vi "Volumes calculation.vi"(1 "Ring":u16(ring) items=["Random", "Regular", "Piecewise regular", "DiRect"], 2 "Params":sgl[][](array[numeric])) -> (0 "Volumes":sgl[](array[numeric]))   [LabVIEW 2018]
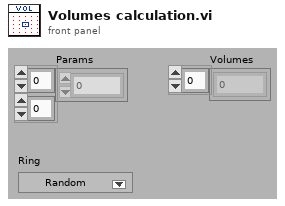
[diagram p1: front panel]
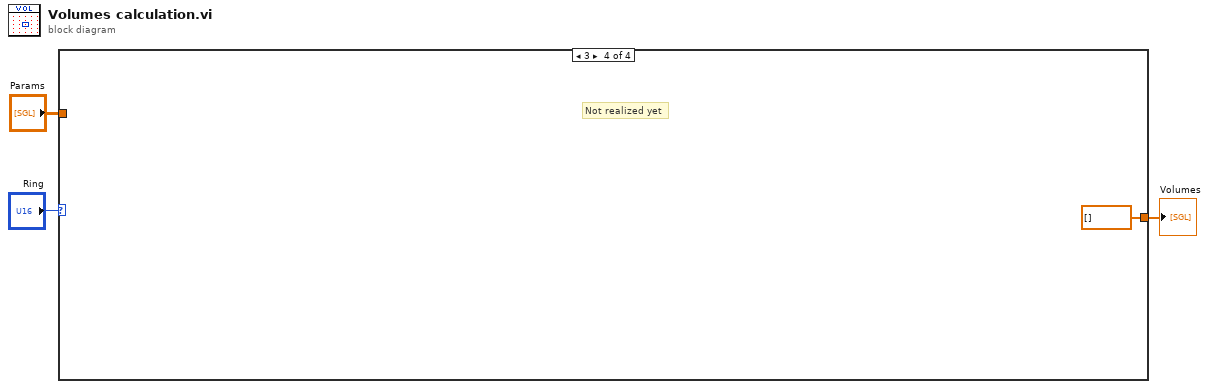
[diagram p0: block diagram]
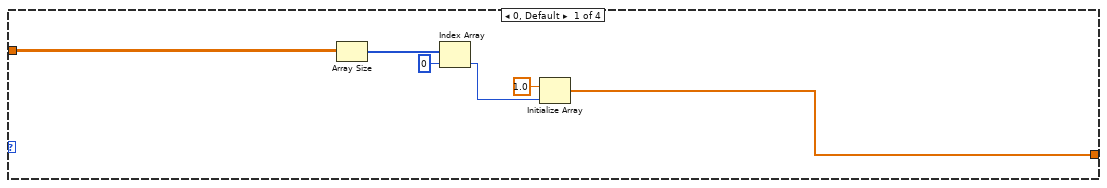
[diagram p2: hidden frame]
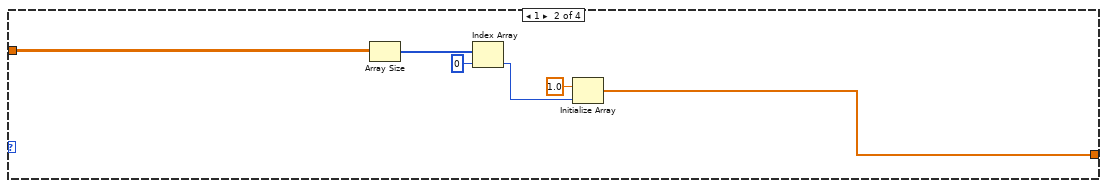
[diagram p3: hidden frame]
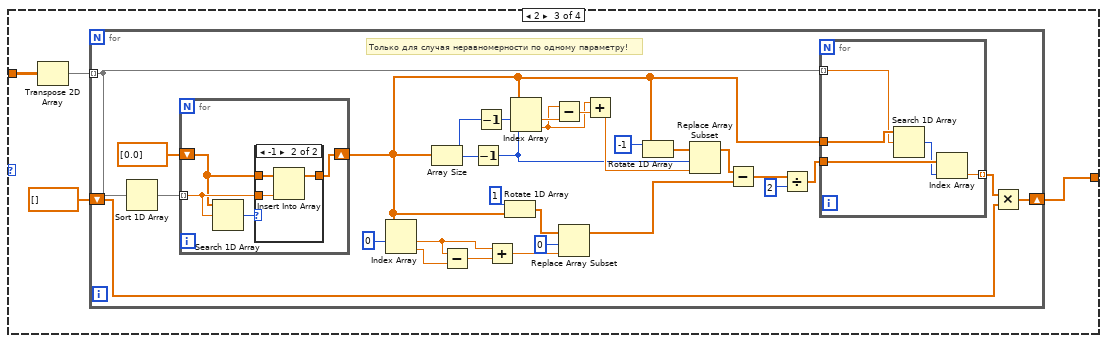
[diagram p4: hidden frame]
diagram:
  n1 = case shown="3" "Ring" {
    tunnel: "Params" -> [w9 w11 w19 _]
    tunnel: [w4 w10 w16 dbl[] []] -> w1
    frame 0, Default {
      n2 = Array Size(array=w9) -> (size(s)=w8:i32[])
      n3 = Index Array(array=w8, index=0) -> (element=w6:i32)
      n4 = Initialize Array(1.0 ("element"), w6) -> (w4:dbl[])
    }
    frame 1 {
      n5 = Array Size(array=w11) -> (size(s)=w12:i32[])
      n6 = Index Array(array=w12, index=0) -> (element=w14:i32)
      n7 = Initialize Array(1.0 ("element"), w14) -> (w10:dbl[])
    }
    frame 2 {
      n8 = Transpose 2D Array(2D array=w19) -> (transposed array=w18:sgl[][])
      n9 = for {
        tunnel: w18 -> [w26] mode=indexing
        shift-right: [w22] -> w16
        shift-left: sgl[] [] -> [w20]
        # "Только для случая неравномерности по одному параметру!"
        n10 = Sort 1D Array(array=w26) -> (sorted array=w25:sgl[])
        n11 = for {
          tunnel: w25 -> [w56] mode=indexing
          shift-right: [w57] -> w24
          shift-left: sgl[] [0.0] ("x-y") -> [w55]
          n12 = Search 1D Array(1D array=w55, element=w56) -> (index of element=w54:i32)  [unwired: 1 in]
          n13 = case shown="-1" w54 {
            tunnel: w56 -> [_ w61]
            tunnel: w55 -> [w58 w60]
            tunnel: [w58 w59] -> w57
            frame 0, Default {
            }
            frame -1 {
              n14 = Insert Into Array(array=w60, new element=w61) -> (w59:sgl[])  [unwired: 1 in]
            }
          }
        }
        n15 = Index Array(array=w24, index #1=0 ("index")) -> (element #1=w41:sgl, element #2=w40:sgl)  [unwired: 1 in]
        n16 = Array Size(array=w24) -> (size(s)=w39:i32)
        n17 = Subtract(x=w41, y=w40) -> (x-y=w42:sgl)
        n18 = Decrement(x=w39) -> (x-1=w31:i32)
        n19 = Decrement(x=w31) -> (x-1=w32:i32)
        n20 = Add(x=w41, y=w42) -> (x+y=w38:sgl)
        n21 = Rotate 1D Array(1:w24, 2:1 ("n")) -> (0:w44:sgl[])
        n22 = Index Array(array=w24, index #1=w32, index #2=w31) -> (element #1=w34:sgl, element #2=w33:sgl)
        n23 = Subtract(x=w33, y=w34) -> (x-y=w43:sgl)
        n24 = Replace Array Subset(array=w44, new element=w38, index=0) -> (w28:sgl[])
        n25 = Add(x=w33, y=w43) -> (x+y=w37:sgl)
        n26 = Rotate 1D Array(1:w24, 2:-1 ("n")) -> (0:w45:sgl[])
        n27 = Replace Array Subset(array=w45, new element=w37, index=w31) -> (w29:sgl[])
        n28 = Subtract(x=w29, y=w28) -> (x-y=w30:sgl[])
        n29 = Divide(x=w30, y=2 ("index")) -> (x/y=w23:sgl[])
        n30 = for {
          tunnel: w26 -> [w50] mode=indexing
          tunnel: w24 -> [w53]
          tunnel: w23 -> [w52]
          tunnel: [w49] -> w21 mode=indexing
          n31 = Search 1D Array(1D array=w53, element=w50) -> (index of element=w51:i32)  [unwired: 1 in]
          n32 = Index Array(array=w52, index=w51) -> (element=w49:sgl)
        }
        n33 = Multiply(x=w21, y=w20) -> (x*y=w22:sgl[])
      }
    }
    frame 3 {
      # "Not realized yet"
    }
  }
  "Volumes" <- w1
